vi "SimpleRamp_Generate_v4.vi"(4 "error in (no error)":errorcluster, 5 "Error Locator":string, 6 "formula":string="sin(10*f)", 7 "Current Variable settings":T1[](array[typedef]), 8 "dt":dbl=1.0, 9 "Points":u32=500) -> (0 "error out":errorcluster, 1 "x values":dbl[](array[numeric]), 2 "y values":dbl[](array[numeric]))   [LabVIEW 2013]
doc: "Right Now this computes the expression on the domain [0,1], but it could be made more general to use actual time units."
uses:
  TypeDefs/Active procedure variables.ctl
  Globals/UserFunctions.vi
  PackedLibraries/LuaEvaluatorAPI.lvlibp
panel:
  # "This computes the expression, where\n\"f\" on the domain [0,1]\nor\n\"t\" varaible is in absolute units."
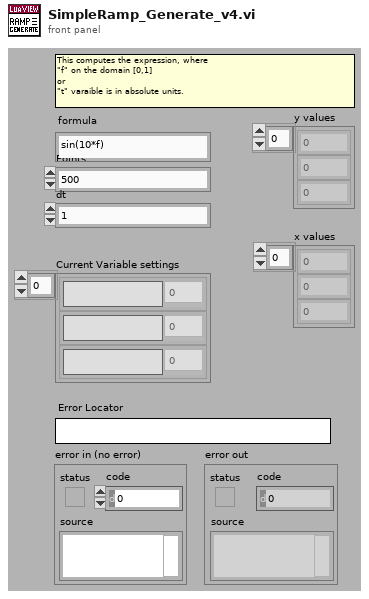
[diagram p1: front panel]
types:
  T1 = typedef "Active procedure variables.ctl" = cluster{"Procedure variable":string, "Value":dbl}
  T2 = enum16{"set", "get", "eval", "assign", "execute", "isvalid", "evaltable"}
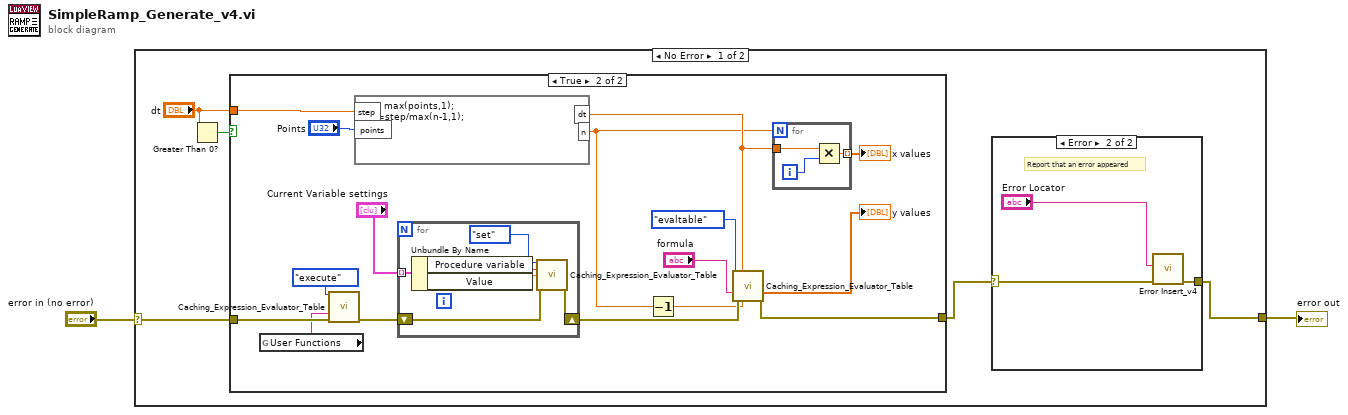
[diagram p0: block diagram]
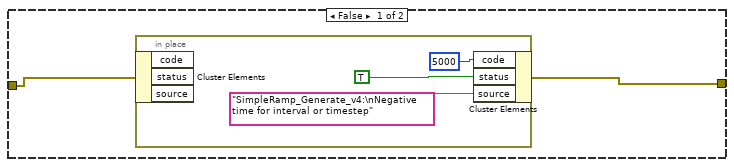
[diagram p3: hidden frame]
diagram:
  n1 = case shown="No Error" "error in (no error)" {
    selector: "error in (no error)" -> [w7 w42]
    tunnel: [w3 w42] -> w1
    frame No Error {
      n2 = Greater Than 0?(x="dt") -> (x > 0?=w5:bool)
      n3 = case shown="True" w5 {
        tunnel: [w12 w31] -> w4
        tunnel: w7 -> [w13 w24]
        tunnel: "dt" -> [_ w20]
        frame False {
          n4 = in-place {
            n5 = in-place-cluster #1(w13) -> ()  [unwired: 3 out]
            n6 = in-place-cluster #1("code"=5000, "status"=TRUE, "source"="SimpleRamp_Generate_v4:\nNegative time for interval or timestep") -> (w12:errorcluster)
          }
        }
        frame True {
          n7 = global read "UserFunctions.vi" "User Functions"() -> (w17:string)
          n8 = call "Caching_Expression_Evaluator_Table.vi"("method"=T2."execute", "expression/scriptlet"=w17, "error in (no error)"=w24) -> ("error out"=w25:errorcluster)  [unwired: 4 in, 8 out]
          n9 = formula code="n = max(points,1);\ndt =step/max(n-1,1);"("points"="Points", "step"=w20) -> ("dt"=w22:dbl, "n"=w19:dbl)
          n10 = for {
            shift-right: [w41] -> w32
            shift-left: w25 -> [w40]
            tunnel: "Current Variable settings" -> [w37] mode=indexing
            n11 = Unbundle By Name(w37) -> ("Procedure variable"=w39:string, "Value"=w38:dbl)
            n12 = call "Caching_Expression_Evaluator_Table.vi"("method"=T2."set", "variable"=w39, "value in"=w38, "error in (no error)"=w40) -> ("error out"=w41:errorcluster)  [unwired: 3 in, 8 out]
          }
          n13 = Decrement(x=w19) -> (x-1=w18:dbl)
          n14 = call "Caching_Expression_Evaluator_Table.vi"("method"=T2."evaltable", "dt (for table)"=w22, "expression/scriptlet"="formula", "error in (no error)"=w32, "steps (for table)"=w18) -> ("table out"=→"y values":dbl[], "error out"=w31:errorcluster)  [unwired: 2 in, 7 out]
          n15 = for {
            N: w19 -> [_]
            tunnel: w22 -> [w35]
            tunnel: [w33] -> w28 mode=indexing
            i -> [w34]
            n16 = Multiply(x=w35, y=w34) -> (x*y=w33:dbl)
          }
          "x values" <- w28
        }
      }
      n17 = case shown="Error" w4 {
        selector: w4 -> [w8 w11]
        tunnel: [w8 w10] -> w3
        frame No Error {
        }
        frame Error {
          # "Report that an error appeared"
          n18 = call "Error Insert_v4.vi"("error in (no error)"=w11, "error message (\"\")"="Error Locator") -> ("error out"=w10:errorcluster)  [unwired: 1 in, 6 out]
        }
      }
    }
    frame Error {
    }
  }
  "error out" <- w1
